vi "Get-action-default-settings.vi"(8 "error in (no error)":errorcluster, 9 "Motor actions":T1, 10 "Action in":refnum<class "Action.lvclass">, 11 "Motor in":refnum<class "Motor-Xaxis.lvclass">) -> (0 "error out":errorcluster, 2 "Action":refnum<class "Action.lvclass">, 3 "Motor out":refnum<class "Motor-Xaxis.lvclass">)   [LabVIEW 2013, in "PowderDeposition.lvlib" / "Motor-Xaxis.lvclass"]
uses:
  Motor-Xaxis.lvclass
  Action/Motor-actions.ctl
  Action/Action.lvclass
  Action/Move-Relative/Move-Relative.lvclass
  Action/Move-Relative/Move-Relative-settings.ctl
  Action/Move-Absolute/Move-Absolute.lvclass
  Action/Move-Absolute/Move-Absolute-settings.ctl
  Action/Home/Home.lvclass
  Action/Substrate/Substrate.lvclass
  Action/Sieve/Sieve.lvclass
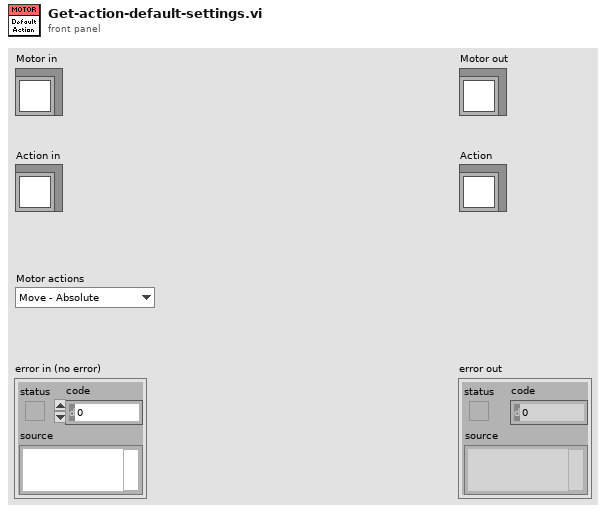
[diagram p1: front panel]
types:
  T1 = typedef "PowderDeposition.lvlib/Action.lvclass/Motor-actions.ctl" = enum16{"Move - Absolute", "Move - Relative", "Move - Timer", "Wait", "Home", "Substrate", "Sieve", "Stop"}
  T2 = typedef "PowderDeposition.lvlib/Move-Relative.lvclass/Move-Relative-settings.ctl" = cluster{"Displacement":dbl, "Speed":dbl, "Direction":enum16{"Clockwise", "Counter-clockwise"}, "Min duration":dbl}
  T3 = typedef "PowderDeposition.lvlib/Move-Absolute.lvclass/Move-Absolute-settings.ctl" = cluster{"Position":dbl, "Speed":dbl, "Min duration":dbl}
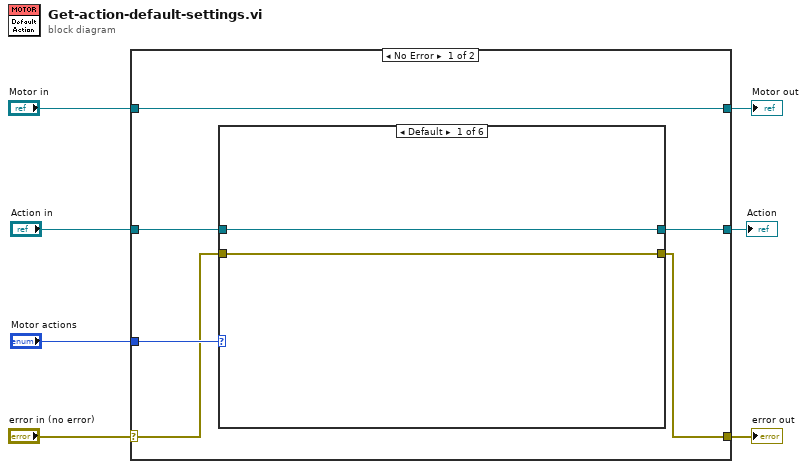
[diagram p0: block diagram]
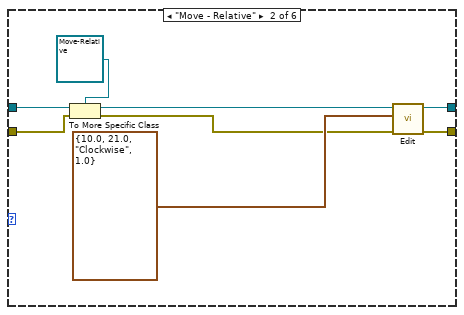
[diagram p2: hidden frame]
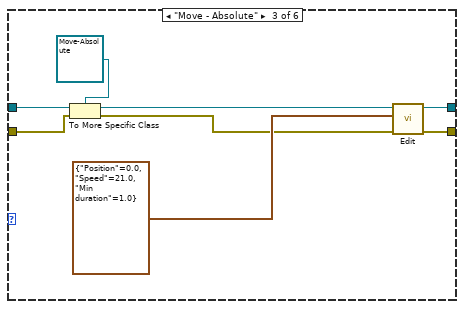
[diagram p3: hidden frame]
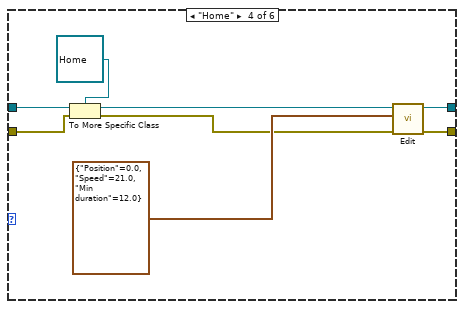
[diagram p4: hidden frame]
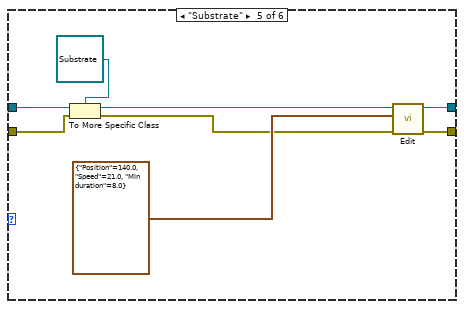
[diagram p5: hidden frame]
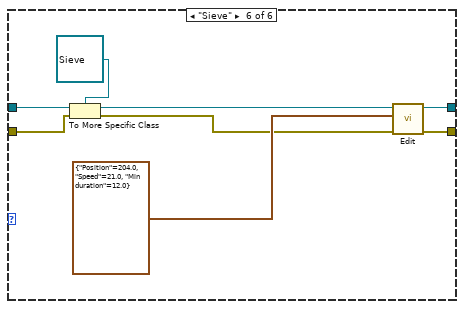
[diagram p6: hidden frame]
diagram:
  n1 = case shown="No Error" "error in (no error)" {
    selector: "error in (no error)" -> [w9 w58]
    tunnel: [w8 w58] -> w6
    tunnel: [w13 w57] -> w4
    tunnel: "Motor in" -> [w13 w57]
    tunnel: "Motor actions" -> [w11 _]
    tunnel: "Action in" -> [w12 w56]
    tunnel: [w10 w56] -> w1
    frame No Error {
      n2 = case shown="Default" w11 {
        tunnel: w12 -> [w15 w23 w31 w39 w47 w55]
        tunnel: [w15 w20 w28 w36 w44 w52] -> w10
        tunnel: [w14 w17 w25 w33 w41 w49] -> w8
        tunnel: w9 -> [w14 w16 w24 w32 w40 w48]
        frame Default {
        }
        frame "Move - Relative" {
          n3 = To More Specific Class(target class=refnum<class "Move-Relative.lvclass"> refnum ("Move-Distance.lvclass"), reference=w23, error in=w16) -> (specific class reference=w21:refnum<class "Move-Relative.lvclass">, error out=w18:errorcluster)
          n4 = call-dynamic "Edit.vi"("error in (no error)"=w18, "Edit dialog"=T2 {"Displacement"=10.0, "Speed"=21.0, "Direction"=enum."Clockwise", "Min duration"=1.0}, "Action in"=w21) -> ("error out"=w17:errorcluster, "Action out"=w20:refnum<class "Move-Relative.lvclass">)  [unwired: 7 in]
        }
        frame "Move - Absolute" {
          n5 = To More Specific Class(target class=refnum<class "Move-Absolute.lvclass"> refnum ("Move-Absolute.lvclass"), reference=w31, error in=w24) -> (specific class reference=w29:refnum<class "Move-Absolute.lvclass">, error out=w26:errorcluster)
          n6 = call-dynamic "Edit.vi"("error in (no error)"=w26, "Edit dialog"=T3 {"Position"=0.0, "Speed"=21.0, "Min duration"=1.0}, "Action in"=w29) -> ("error out"=w25:errorcluster, "Action out"=w28:refnum<class "Move-Absolute.lvclass">)  [unwired: 7 in]
        }
        frame "Home" {
          n7 = To More Specific Class(target class=refnum<class "Home.lvclass"> refnum ("Home.lvclass"), reference=w39, error in=w32) -> (specific class reference=w37:refnum<class "Home.lvclass">, error out=w34:errorcluster)
          n8 = call-dynamic "Edit.vi"("error in (no error)"=w34, "Edit dialog"=T3 {"Position"=0.0, "Speed"=21.0, "Min duration"=12.0}, "Action in"=w37) -> ("error out"=w33:errorcluster, "Action out"=w36:refnum<class "Home.lvclass">)  [unwired: 7 in]
        }
        frame "Substrate" {
          n9 = To More Specific Class(target class=refnum<class "Substrate.lvclass"> refnum ("Substrate.lvclass"), reference=w47, error in=w40) -> (specific class reference=w45:refnum<class "Substrate.lvclass">, error out=w42:errorcluster)
          n10 = call-dynamic "Edit.vi"("error in (no error)"=w42, "Edit dialog"=T3 {"Position"=140.0, "Speed"=21.0, "Min duration"=8.0}, "Action in"=w45) -> ("error out"=w41:errorcluster, "Action out"=w44:refnum<class "Substrate.lvclass">)  [unwired: 7 in]
        }
        frame "Sieve" {
          n11 = To More Specific Class(target class=refnum<class "Sieve.lvclass"> refnum ("Sieve.lvclass"), reference=w55, error in=w48) -> (specific class reference=w53:refnum<class "Sieve.lvclass">, error out=w50:errorcluster)
          n12 = call-dynamic "Edit.vi"("error in (no error)"=w50, "Edit dialog"=T3 {"Position"=204.0, "Speed"=21.0, "Min duration"=12.0}, "Action in"=w53) -> ("error out"=w49:errorcluster, "Action out"=w52:refnum<class "Sieve.lvclass">)  [unwired: 7 in]
        }
      }
    }
    frame Error {
    }
  }
  "error out" <- w6
  "Motor out" <- w4
  "Action" <- w1
